vi "eWriteName Loop.vi"() -> (0 "error out":errorcluster)   [LabVIEW 2020]
panel:
  in  "Value":dbl=2.5 format="%.6f"
  in  "Name":string="DAC0"
  in  "stop":bool
  in  "Interval [ms]":i32=500
  out "Error String":string
  out "ConnectionType Out":i32
  out "DeviceType Out":i32
  in  "Identifier":string="LJM_idANY"
  in  "ConnectionType":string="LJM_ctANY"
  in  "DeviceType":string="LJM_dtANY"
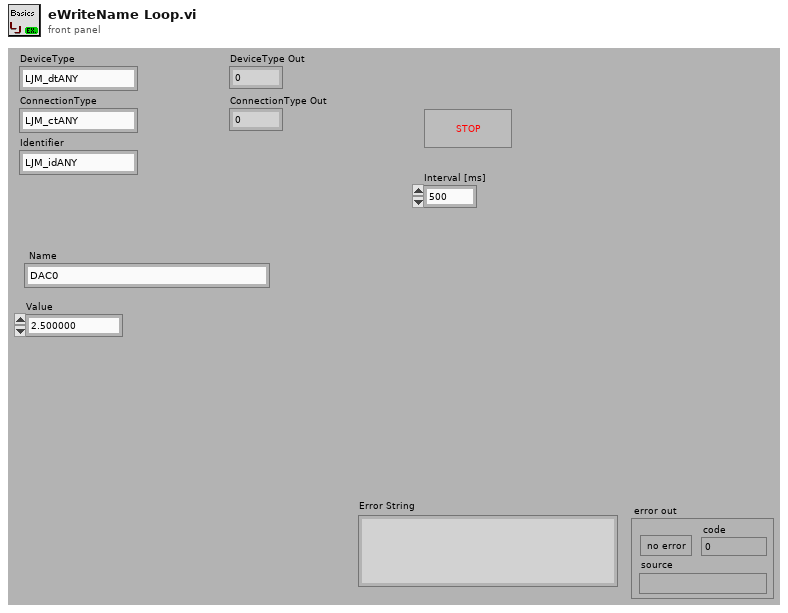
[diagram p1: front panel]
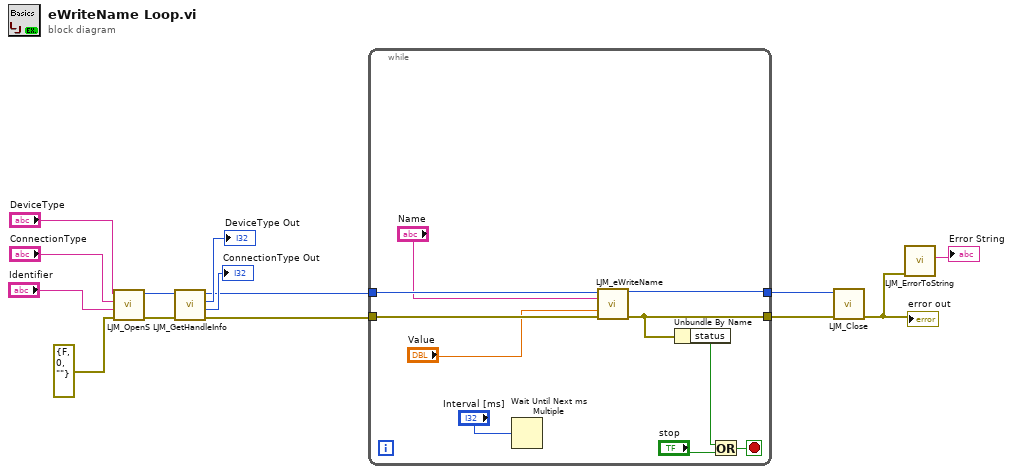
[diagram p0: block diagram]
diagram:
  n1 = call "LJM_OpenS.vi"("error in"=errorcluster {"status"=FALSE, "code"=0, "source"=""} ("error in (no error)"), "Identifier"="Identifier", "ConnectionType"="ConnectionType", "DeviceType"="DeviceType") -> ("error out"=w13:errorcluster, "Handle"=w12:i32)  [unwired: 6 in]
  n2 = call "LJM_GetHandleInfo.vi"("error in"=w13, "Handle In"=w12) -> ("error out"=w1:errorcluster, "ConnectionType"=→"ConnectionType Out":i32, "DeviceType"=→"DeviceType Out":i32, "Handle Out"=w2:i32)  [unwired: 2 in, 4 out]
  n3 = while {
    tunnel: w1 -> [w24]
    tunnel: [w17] -> w4
    tunnel: w2 -> [w23]
    tunnel: [w18] -> w3
    stop <- w21 stop-if-true
    n4 = Wait Until Next ms Multiple(millisecond multiple="Interval [ms]") -> ()  [unwired: 1 out]
    n5 = call "LJM_eWriteName.vi"("Handle In"=w23, "Name"="Name", "Value"="Value", "error in"=w24) -> ("Handle Out"=w18:i32, "error out"=w17:errorcluster)  [unwired: 10 in]
    n6 = Unbundle By Name(w17) -> ("status"=w20:bool)
    n7 = Or(x=w20, y="stop") -> (x .or. y?=w21:bool)
  }
  n8 = call "LJM_Close.vi"("error in"=w4, "Handle"=w3) -> ("error out"=w6:errorcluster)  [unwired: 9 in]
  "error out" <- w6
  n9 = call "LJM_ErrorToString.vi"("error in"=w6) -> ("String"=→"Error String":string)  [unwired: 10 in]
